vi "Dashboard Main.vi.BASE.11652.vi"() -> ()   [LabVIEW 2014]
uses:
  AutonModes.ctl
  <vilib>/event_ctls.llb/eventvkey.ctl
  <vilib>/Rock Robotics/WPI/Dashboard/WPI_DashboardLogging Global.vi
  <vilib>/Rock Robotics/Network Tables/SD Write String.vi
  <vilib>/Rock Robotics/Network Tables/SD Read String.vi
  <vilib>/Utility/config.llb/Write Key (String).vi
  <vilib>/Utility/config.llb/Write Key (I32).vi
  <vilib>/Utility/config.llb/NI_LVConfig.lvlib
panel:
  in  "TCP":refnum<k5>
  in  "Rec Mode":enum32{"Stop", "Record", "Playback"}(radio)
  in  "Vision":u16(ring) items=["Camera Off", "USB Camera SW", "USB Camera HW", "IP Camera"]
  out "Camera IP":string
  out "Image Message":string="Timeout in Camera Communications"
  in  "Dashboard Tab":T1(tab)
  in  "Camera Settings":T2={"Frame Rate"=30, "Compression"=30, "Size"=1} {"Frame Rate" scale=1.0..30.0; "Size" items=["640x480", "320x240", "160x120"]}
  out "MotorChart R":cluster{"Numeric":dbl, "Numeric":dbl}(graph)
  out "MotorChart L":T3(graph)
  out "MotorSliders R":cluster{"MotorSlide1":dbl, "MotorSlide2":dbl} {"MotorSlide2" scale=-1.0..1.0 scale format="%#_2e"; "MotorSlide1" scale=-1.0..1.0 scale format="%#_2e"}
  out "MotorSliders L":T4 {"MotorSlide4 2" scale=0.0..14.0 scale format="%#_2e"; "MotorSlide2" scale=-1.0..1.0 scale format="%#_2e"; "MotorSlide1" scale=-1.0..1.0 scale format="%#_2e"}
  out "Gyro":dbl(knob) scale=0.0..360.0
  out "JS1 Z":dbl(slide) scale=-1.0..1.0 scale format="%#_2e"
  out "JS1 Graph":cluster{"X":dbl, "Y":dbl}[](graph)
  out "JS1 Buttons":T5
  out "JS2 Z":dbl(slide) scale=-1.0..1.0 scale format="%#_2e"
  out "JS2 Graph":cluster{"X":dbl, "Y":dbl}[](graph)
  out "JS2 Buttons":T5
  out "Mode":T6(ring)=enum."Auto Disabled"
  in  "DB Camera Config":bool
  out "fps":dbl format="%#.1g"
  out "Mbps":dbl format="%#.1g"
  out "Mbps 2":bool
  in  "Open Config File":bool
  in  "Auton Mode":T7
  in  "Path to Auton Configs":path=path "C:/AutoConfig"
  out "Current Overdraw":bool
  out "Current":T8(graph)
  in  "DB/String 9":string
  in  "DB/String 8":string
  in  "DB/String 7":string
  in  "DB/String 6":string
  in  "DB/String 5":string
  in  "DB/String 4":string
  in  "DB/String 3":string
  in  "DB/String 2":string
  in  "DB/String 1":string
  in  "DB/String 0":string
  in  "DB/Slider 0":dbl(slide) scale=0.0..5.0
  in  "DB/Slider 1":dbl(slide) scale=0.0..5.0
  in  "DB/Slider 2":dbl(slide) scale=0.0..5.0
  in  "DB/Slider 3":dbl(slide) scale=0.0..5.0
  out "DB/LED 3":bool
  out "DB/LED 2":bool
  out "DB/LED 1":bool
  out "DB/LED 0":bool
  in  "DB/Button 3":bool
  in  "DB/Button 2":bool
  in  "DB/Button 1":bool
  in  "DB/Button 0":bool caption="New Name"
  in  "Test Slider":dbl(slide) scale=0.0..100.0 scale format="%#_3g"
  in  "On/Off":bool caption="Solenoid"
  in  "Test Name":u16(ring) items=["Select the test to run...", "Example Test", "-------------------------------", "List of tests is built in robot code.", "Replace with your own automated tests."]
  in  "Test Tree":string(tree)
  in  "Motor":cluster{"Value":dbl, "Enable":bool} {"Value" scale=-1.0..1.0 scale format="%#_3g"}
  out "Progress":T9 {"Test Progress" scale=0.0..100.0}
  in  "Rev/Fwd":cluster{"Forward":bool, "Reverse":bool}
  in  "Test Ring":u16(ring) items=["Monochrome", "Color"]
  in  "Listbox":i32(listbox)
  out "Tree":string(tree)
  out "Camera Image":T10(plugin-control)
  out "Boolean":bool
  # "Left"
  # "Front"
  # "Right"
  # "Battery"
  # "This tab is a great place for autonomous settings and robot-specific values.\nPlace controls and indicators inside this tab and match name to\nDashboard Variables on robot. You can also delete this comment."
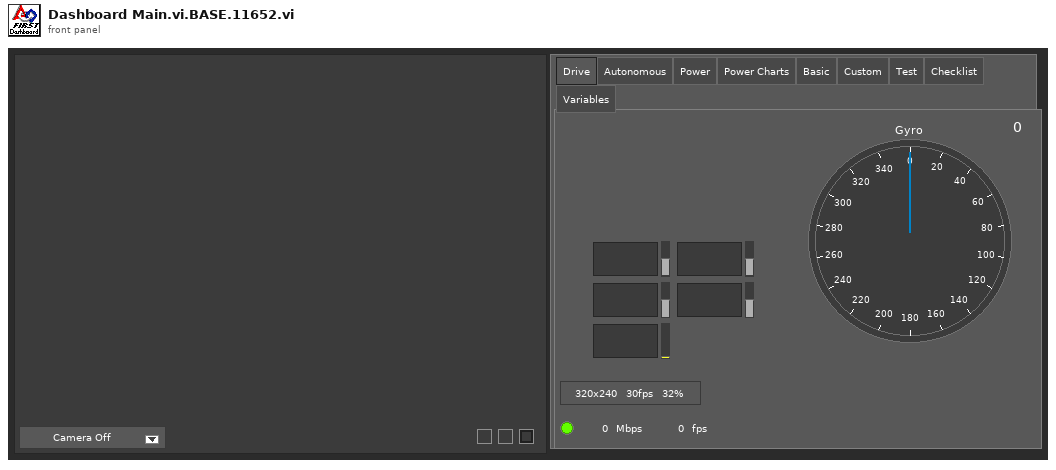
[diagram p1: front panel]
types:
  T1 = enum32{"Drive", "Autonomous", "Power", "Power Charts", "Basic", "Custom", "Test", "Checklist", "Variables"}
  T2 = cluster{"Frame Rate":i32, "Compression":i32, "Size":u16}
  T3 = cluster{"Numeric":dbl, "Numeric":dbl, "Battery V":dbl}
  T4 = cluster{"MotorSlide1":dbl, "MotorSlide2":dbl, "MotorSlide4 2":dbl}
  T5 = cluster{bool, bool, bool, bool, bool, bool, bool, bool, bool, bool, bool, bool}
  T6 = enum8{"Tele-Op Disabled", "Tele-Op Enabled", "Auto Disabled", "Auto Enabled", "Test Disabled", "Test Enabled", "Disconnected", "No Code", "E-Stop"}
  T7 = typedef "AutonModes.ctl" = enum32{"Sit Still", "Go Get That Tote!", "Custom 1", "Custom 2", "FromLandfill", "CanGrab"}
  T8 = cluster{"Numeric":dbl, "Numeric":dbl, "Numeric":dbl, "Numeric":dbl, "Numeric":dbl}
  T9 = cluster{"Test Progress":u8, "Test Progress Text":string}
  T10 = typedef "IMAQ Image.ctl" = refnum<image>
  T11 = enum32{"Drive", "Basic", "Custom", "Test", "Checklist", "Variables"}
  T12 = typedef "Image Type" = u32
  T13 = cluster{"Camera Image":refnum<vi>, "Dashboard Tab":refnum<vi>, "Boolean":refnum<vi>, "Vision":refnum<vi>, "Rec Mode":refnum<vi>, "Test Slider":refnum<vi>, "On/Off ":refnum<vi>, "Test Ring":refnum<vi>, "Rev/Fwd":refnum<vi>, "Test Name":refnum<vi>, "Motor":refnum<vi>, "Progress":refnum<vi>, "CheckList":refnum<vi>, "Tree":refnum<vi>, "Test Tree":refnum<vi>}
  T14 = enum16{"open", "replace", "create", "open or create", "replace or create", "replace or create with confirmation"}
  T15 = cluster{"Error Strings":string, "Disable Counts":cluster{u16, u16}, "Rail Faults":cluster{u16, u16, u16}, "Robot IP":string, "DB Mode":u8, "Event Info":cluster{"Name":string, "Type":u8, "Number":u16, "Replay":u8}, "Camera Addr":string}
  T16 = cluster{"Storage":cluster{"Disk Free":u64, "RAM Block":u32, "RAM free":u32}, "CPU Utilization":cluster{"CPU % ISR":sgl, "CPU % Time Crit":sgl, "CPU % Timed Str":sgl, "CPU % High":sgl, "CPU % Above":sgl, "CPU % Normal":sgl, "CPU % Low":sgl}, "CAN":cluster{"% Bus Utilization":sgl, "Bus Off Cnt":u32, "TX_FIFO Full Cnt":u32, "Receive Error Cnt":u8, "Transmit Error Cnt":u8}, "HID":cluster{"HID Outputs":u32, "Rumble Low":u16, "Rumble High":u16}[]}
  T17 = cluster{"Status bits":cluster{"Test Mode":bool, "Autonomous":bool, "Enabled":bool, "Code Start":bool, "Brownout":bool, "Reserved 2":bool, "Reserved 3":bool, "E-Stop":bool}, "Code Trace":cluster{"Disabled":bool, "TeleOp":bool, "Auto":bool, "Test":bool}, "Controller Type":enum16{"unknown", "cRIO", "roboRio"}, "Code?":enum16{"unknown", "noCode", "code"}, "Battery V":dbl}
  T18 = cluster{"Control Bits":cluster{"TestMode":bool, "Autonomous":bool, "Enabled":bool, "FMS Present":bool, bool, bool, bool, "E-Stop":bool}, "Team Station ":u8, "Countdown":sgl, "Joystick Values":cluster{"Axes":dbl[], "Buttons":bool[], "POVs":i16[]}[]}
  T19 = cluster{"Axes":dbl[], "Buttons":bool[], "POVs":i16[]}[]
  T20 = cluster{"Axes":dbl[], "Buttons":bool[], "POVs":i16[]}
  T21 = cluster{"Buttons[0]":bool, "Buttons[1]":bool, "Buttons[2]":bool, "Buttons[3]":bool, "Buttons[4]":bool, "Buttons[5]":bool, "Buttons[6]":bool, "Buttons[7]":bool, "Buttons[8]":bool, "Buttons[9]":bool, "Buttons[10]":bool, "Buttons[11]":bool}
  T22 = typedef "NI_LVConfig.lvlib/Config Data RefNum.ctl" = refnum<k1>
  T23 = cluster{"Operation":enum16{"Update", "Clear"}, "Color Box":u32}[]
  T24 = typedef "eventvkey.ctl" = enum16{"ASCII", "Enter", "Return", "Shift", "Ctrl", "Alt", "Cmd", "Opt", "Caps", "NumLock", "Clear", "Break", "Up", "Down", "Left", "Right", "Insert", "Delete", "Home", "End", "PageUp", "PageDown", "Escape", "Help", "Pause", "ScrollLock", "F1", "F2", "F3", "F4", "F5", "F6", "F7", "F8", "F9", "F10", "F11", "F12", "F13", "F14", "F15", "F16", "F17", "F18", "F19", "F20", "F21", "F22", "F23", "F24", "Play", "VolumeUp", "VolumeDown", "Mute", "Two Byte Char"}
  T25 = cluster{"Image Size":bool, "Image Type":bool, "Pixel Value":bool, "ROI Information":bool, "Zoom Factor":bool}
  T26 = enum8{"Enabled", "Disabled", "Disabled and Grayed Out"}
  T27 = cluster{"Operation":enum16{"Update", "Clear"}, "Color Box":u32}
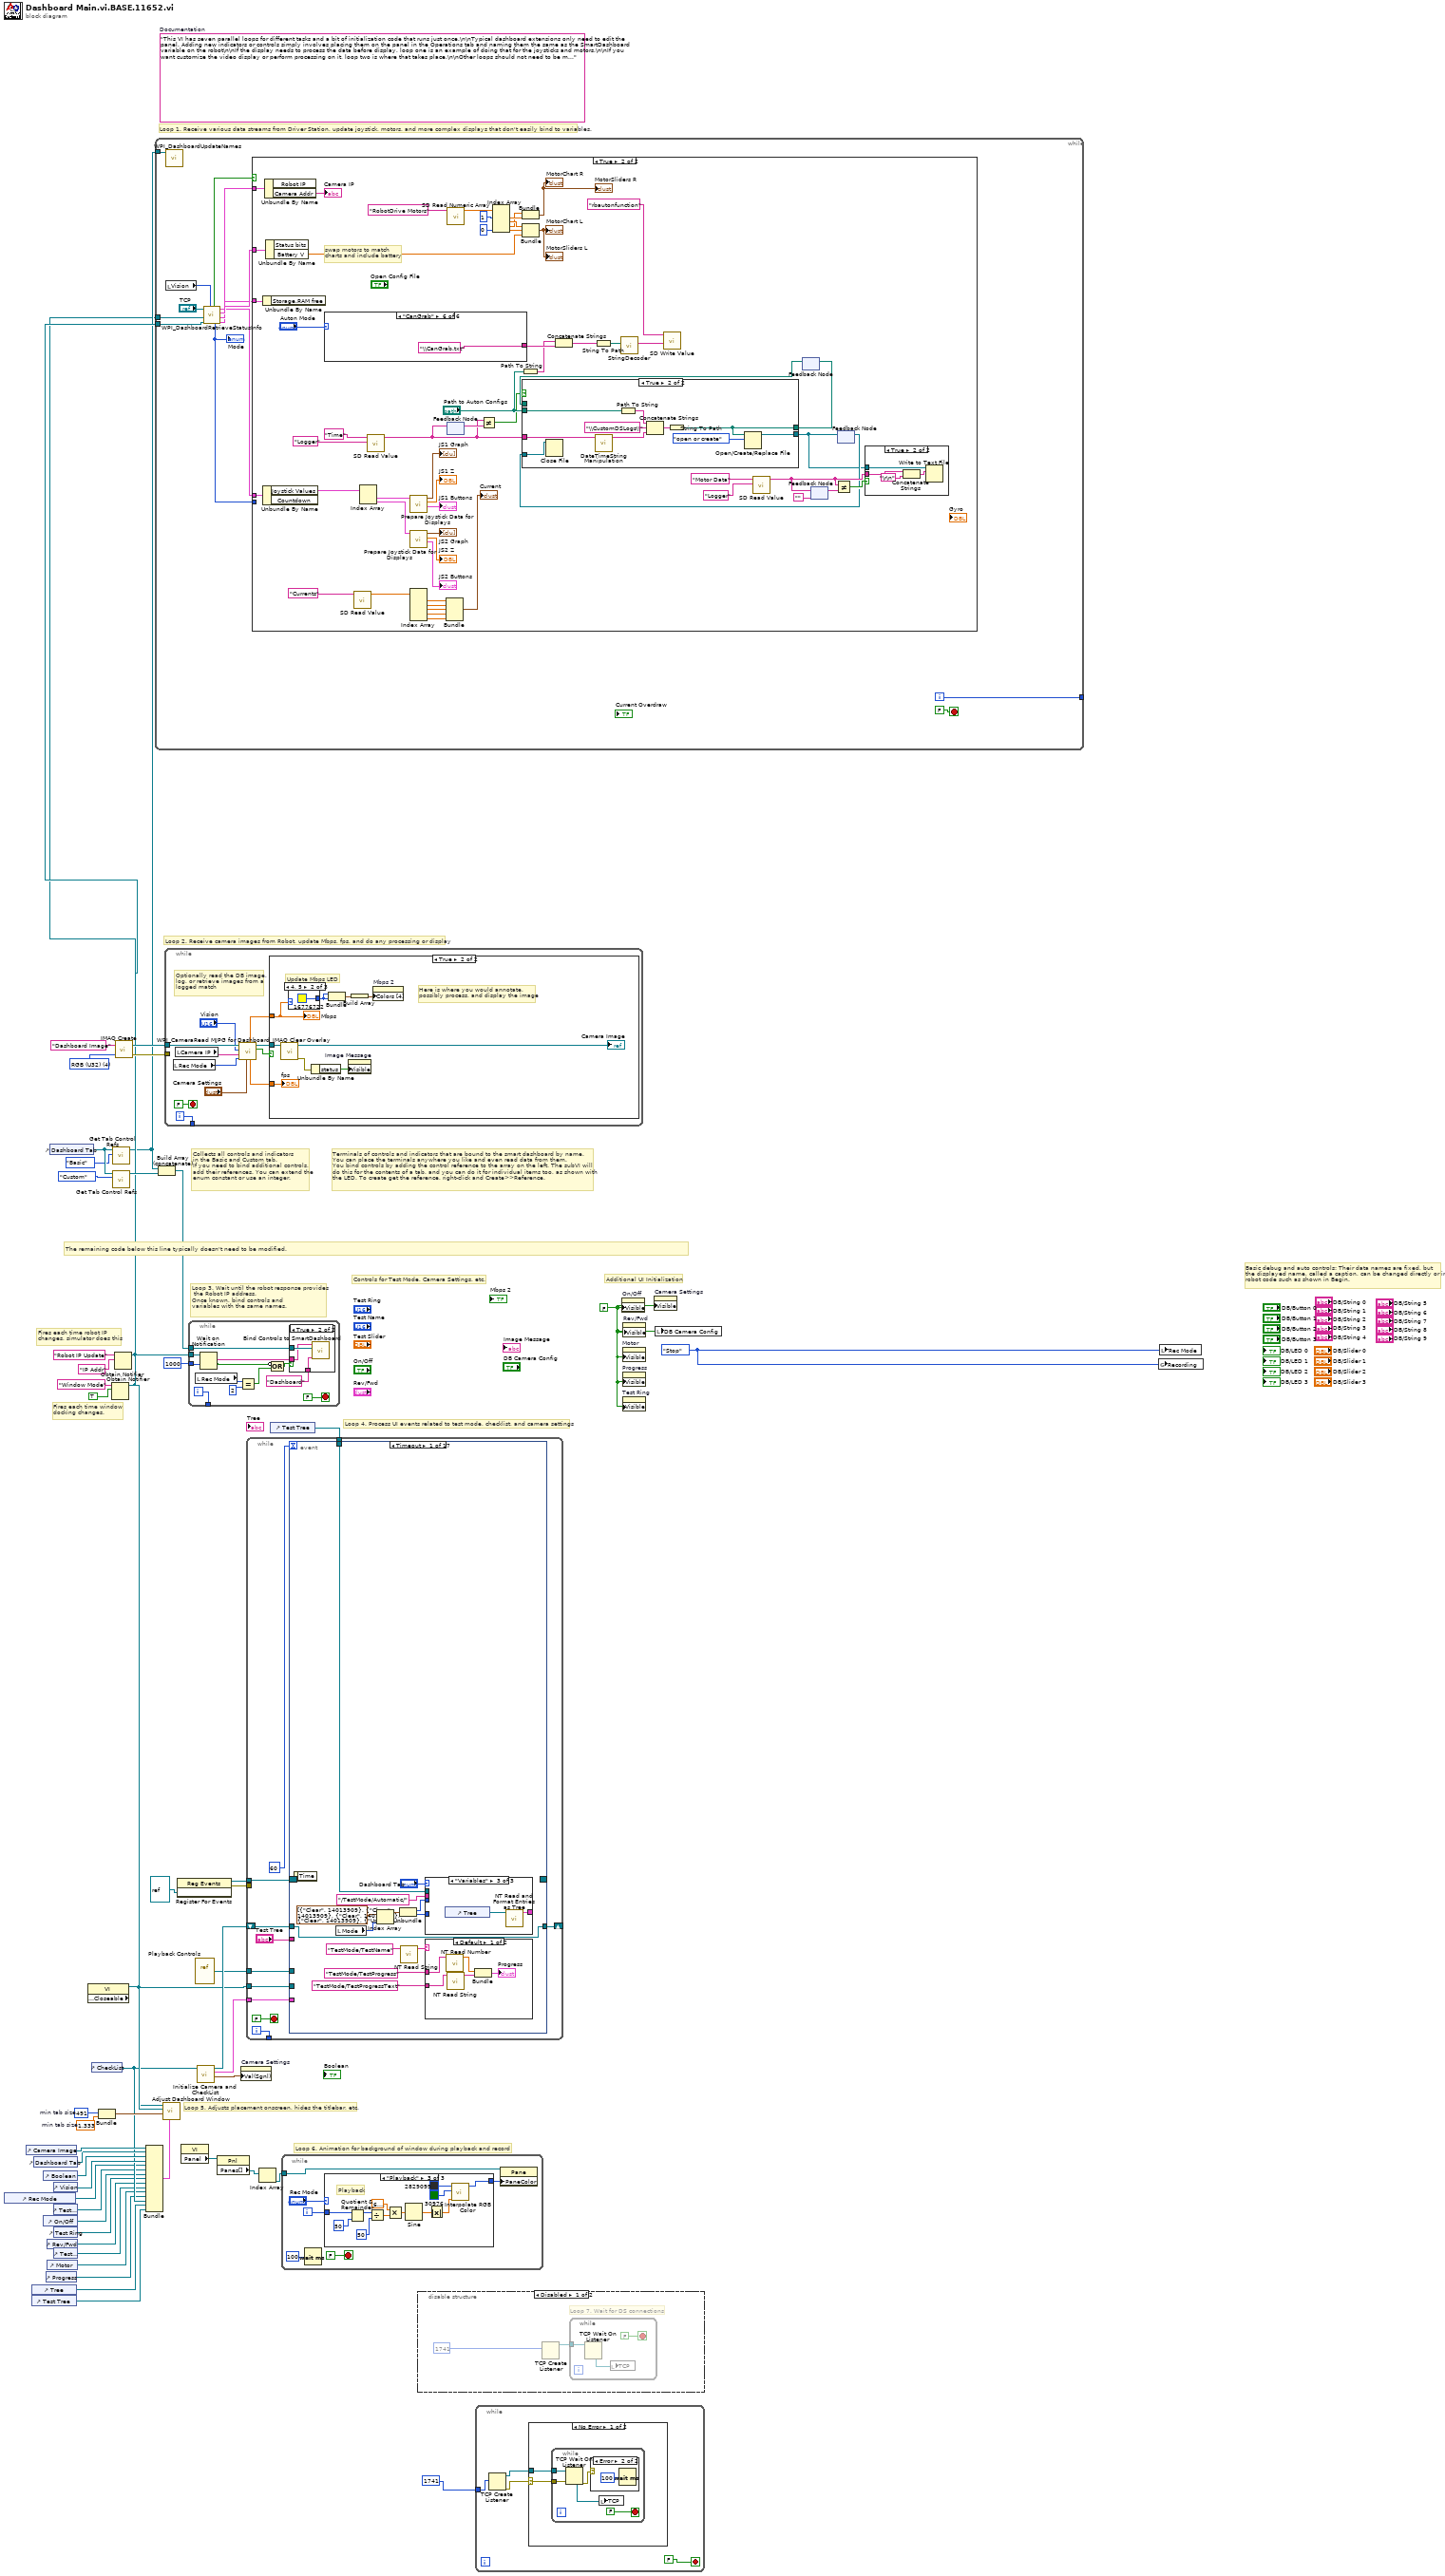
[diagram p0: block diagram]
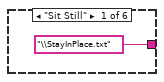
[diagram p8: hidden frame]
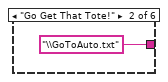
[diagram p9: hidden frame]
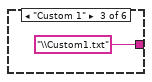
[diagram p10: hidden frame]
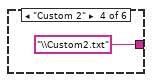
[diagram p11: hidden frame]
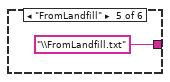
[diagram p12: hidden frame]
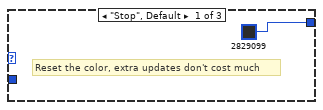
[diagram p13: hidden frame]
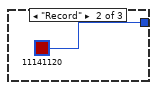
[diagram p14: hidden frame]
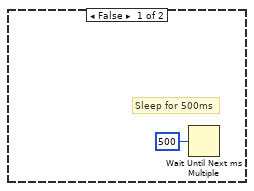
[diagram p16: hidden frame]
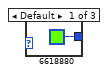
[diagram p17: hidden frame]
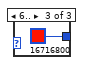
[diagram p18: hidden frame]
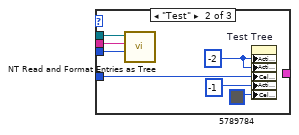
[diagram p20: hidden frame]
diagram:
  w23 = 491  # min tab size
  w22 = 1.333  # min tab size
  w31 = enum32{"Stop", "Record", "Playback"}."Stop" ("Rec Mode")
  w5 = FALSE ("Visible")
  (unwired) "This VI has seven parallel loops for different tasks and a bit of initialization code that runs just once.\n\nTypical dashboard extensions only need to edit the panel. Adding new indicators or controls simply involves placing them on the panel in the Operations tab and naming them the same as the SmartDashboard variable on the robot\n\nIf the display needs to process the data before display, loop one is an example of doing that for the joysticks and motors.\n\nIf you want customize the video display or perform processing on it, loop two is where that takes place.\n\nOther loops should not need to be modified. They are pretty standard, and document the task they perform."  # Documentation
  w51 = T12 4 items=["Grayscale (U8)", "Grayscale (I16)", "Grayscale (SGL)", "Complex (CSG)", "RGB (U32)", "HSL (U32)", "RGB (U64)"] ("Image Type")
  # "Basic debug and auto controls: Their data names are fixed, but\nthe displayed name, called a caption, can be changed directly or in\nrobot code such as shown in Begin."
  # "Controls for Test Mode, Camera Settings, etc."
  # "Additional UI Initialization"
  # "Loop 6. Animation for background of window during playback and record"
  # "Fires each time robot IP\nchanges, simulator does this"
  # "Fires each time window\ndocking changes."
  # "Collects all controls and indicators\nin the Basic and Custom tab.\nIf you need to bind additional controls,\nadd their references. You can extend the\nenum constant or use an integer."
  # "The remaining code below this line typically doesn't need to be modified."
  # "Loop 4. Process UI events related to test mode, checklist, and camera settings"
  # "Terminals of controls and indicators that are bound to the smart dashboard by name.\nYou can place the terminals anywhere you like and even read data from them.\nYou bind controls by adding the control reference to the array on the left. The subVI will\ndo this for the contents of a tab, and you can do it for individual items too, as shown with\nthe LED. To create get the reference, right-click and Create>>Reference."
  # "Loop 3. Wait until the robot response provides\n the Robot IP address.\nOnce known, bind controls and\nvariables with the same names."
  # "Loop 5. Adjusts placement onscreen, hides the titlebar, etc."
  # "Loop 1. Receive various data streams from Driver Station, update joystick, motors, and more complex displays that don't easily bind to variables."
  # "Loop 2. Receive camera images from Robot, update Mbps, fps, and do any processing or display"
  n1 = control-ref of="Rec Mode"() -> (w11:refnum<vi>)
  n2 = control-ref of="Camera Image"() -> (w26:refnum<vi>)
  n3 = control-ref of="Tree"() -> (w15:refnum<vi>)
  n4 = control-ref of="Test Tree"() -> (w14:refnum<vi>)
  n5 = control-ref of="Dashboard Tab"() -> (w25:refnum<vi>)
  n6 = control-ref of="Boolean"() -> (w20:refnum<vi>)
  n7 = control-ref of="On/Off"() -> (w9:refnum<vi>)
  n8 = control-ref of="Progress"() -> (w6:refnum<vi>)
  n9 = control-ref of="Rev/Fwd"() -> (w7:refnum<vi>)
  n10 = control-ref of="Motor"() -> (w12:refnum<vi>)
  n11 = control-ref of="Dashboard Tab"() -> (w29:refnum<vi>)
  n12 = control-ref of="Test Slider"() -> (w10:refnum<vi>)
  n13 = control-ref of="Vision"() -> (w24:refnum<vi>)
  n14 = control-ref of="Test Ring"() -> (w8:refnum<vi>)
  n15 = control-ref of="Test Name"() -> (w13:refnum<vi>)
  n16 = property class="VI" props=["Front Panel.Closeable"]() -> (reference out=w30:refnum<vi>)  [unwired: 2 in, 2 out]
  n17 = control-ref of="CheckList"() -> (w16:refnum<vi>)
  n18 = Bundle("min tab size"=w23, "min tab size"=w22) -> (w21:cluster{"min tab size":i32, "min tab size":dbl})  [unwired: 1 in]
  n19 = Obtain Notifier(name (unnamed)="Window Mode", notification data type=TRUE) -> (notifier out=w2:refnum<notifier>)  [unwired: 2 in, 2 out]
  n20 = call <vilib>:"Get Tab Control Refs.vi"("Page Index"=T11."Basic" ("Dashboard Tab"), "TabControl in"=w29) -> ("ControlsOnPage"=w3:refnum<vi>[])  [unwired: 9 in]
  n21 = call <vilib>:"Get Tab Control Refs.vi"("Page Index"=T11."Custom" ("Dashboard Tab"), "TabControl in"=w29) -> ("ControlsOnPage"=w28:refnum<vi>[])  [unwired: 9 in]
  n22 = Obtain Notifier(name (unnamed)="Robot IP Update", notification data type="IP Addr" ("name (unnamed)")) -> (notifier out=w4:refnum<notifier>)  [unwired: 2 in, 2 out]
  n23 = call "IMAQ Create"("Image Name"="Dashboard Image", "Image Type"=w51) -> ("New Image"=w49:T10, "error out"=w48:errorcluster)  [unwired: 2 in, 1 out]
  n24 = Bundle("Camera Image"=w26, "Dashboard Tab"=w25, "Boolean"=w20, "Vision"=w24, "Rec Mode"=w11, "Test Slider"=w10, "On/Off"=w9, "Test Ring"=w8, "Rev/Fwd"=w7, "Test Name"=w13, "Motor"=w12, "Progress"=w6, "CheckList"=w16, "Tree"=w15, "Test Tree"=w14) -> (w17:T13)  [unwired: 1 in]
  n25 = while {
    tunnel: [w63] -> _
    tunnel: w4 -> [w57]
    tunnel: w3 -> [w56]
    tunnel: w2 -> [w52]
    i -> [w63]
    stop <- FALSE stop-if-true
    n26 = call <vilib>:"WPI_DashboardUpdateNames.vi"("Controls on Tab"=w56) -> ()  [unwired: 11 in]
    n27 = local read "Vision"() -> (w54:u16)
    n28 = call <vilib>:"WPI_DashboardRetrieveStatusInfo.vi"("Vision"=w54, "Binding Refnum"=w57, "Window Mode Notifier"=w52, "TCP Cnx"="TCP") -> ("Power and Errors"=w58:T15, "Robot Metrics"=w61:T16, "Status Info"=w62:T17, "Control Info"=w59:T18, "Robot Mode"=w55:T6, "Process?"=w60:bool)  [unwired: 2 in]
    "Mode" <- w55
    n29 = case shown="True" w60 {
      tunnel: w62 -> [_ w120]
      tunnel: w61 -> [_ w119]
      tunnel: w59 -> [_ w118]
      tunnel: w58 -> [_ w117]
      tunnel: w55 -> [_ _]
      frame False {
      }
      frame True {
        # "swap motors to match\ncharts and include battery"
        n30 = Unbundle By Name(w119) -> ()  [unwired: 1 out]
        n31 = Unbundle By Name(w118) -> ("Joystick Values"=w105:T19)  [unwired: 1 out]
        n32 = Unbundle By Name(w117) -> ("Camera Addr"=→"Camera IP":string)  [unwired: 1 out]
        n33 = Unbundle By Name(w120) -> ("Battery V"=w106:dbl)  [unwired: 1 out]
        n34 = case shown="\"CanGrab\"" "Auton Mode" {
          tunnel: ["\\StayInPlace.txt" "\\GoToAuto.txt" "\\Custom1.txt" "\\Custom2.txt" "\\FromLandfill.txt" "\\CanGrab.txt"] -> w84
          frame "Sit Still" {
          }
          frame "Go Get That Tote!" {
          }
          frame "Custom 1" {
          }
          frame "Custom 2" {
          }
          frame "FromLandfill" {
          }
          frame "CanGrab" {
          }
        }
        n35 = call-poly <vilib>:"SD Read Value.vi"("Name"="Currents") -> ("Numeric Array"=w91:dbl[])  [unwired: 8 in, 2 out]
        n36 = Index Array(array=w105) -> (element #1=w104:T20, element #2=w99:T20)  [unwired: 2 in]
        n37 = call-poly <vilib>:"SD Read Value.vi"("Table Prefix"="Logger", "Name"="Time") -> ("String"=w67:string)  [unwired: 7 in, 2 out]
        n38 = call "Prepare Joystick Data for Displays.vi"("Joystick Values"=w104) -> ("Buttons"=→"JS1 Buttons":T21, "Z Axis"=→"JS1 Z":dbl, "Cartesian Data"=→"JS1 Graph":cluster{"X axis":dbl, "X axis":dbl}[])  [unwired: 8 in]
        n39 = call "Prepare Joystick Data for Displays.vi"("Joystick Values"=w99) -> ("Buttons"=→"JS2 Buttons":T21, "Z Axis"=→"JS2 Z":dbl, "Cartesian Data"=→"JS2 Graph":cluster{"X axis":dbl, "X axis":dbl}[])  [unwired: 8 in]
        n40 = Index Array(array=w91) -> (element #1=w90:dbl, element #2=w89:dbl, element #3=w88:dbl, element #4=w87:dbl, element #5=w86:dbl)  [unwired: 5 in]
        n41 = Bundle("Numeric"=w90, "Numeric"=w89, "Numeric"=w88, "Numeric"=w87, "Numeric"=w86) -> (→"Current":T8)  [unwired: 1 in]
        n42 = call <vilib>:"SD Read Numeric Array.vi"("Name"="RobotDrive Motors") -> ("Numeric Array"=w108:dbl[])  [unwired: 8 in, 2 out]
        n43 = feedback #1() -> (w69:string)  [unwired: 1 in]
        n44 = feedback-in #1(w67) -> ()
        n45 = Not Equal?(x=w67, y=w69) -> (x != y?=w68:bool)
        n46 = Index Array(array=w108, index #1=1, index #4=0) -> (element #1=w112:dbl, element #2=w113:dbl, element #3=w111:dbl, element #4=w116:dbl)  [unwired: 2 in]
        n47 = Path To String(path="Path to Auton Configs") -> (string=w83:string)
        n48 = Bundle("Numeric"=w111, "Numeric"=w112) -> (→"MotorChart R" →"MotorSliders R":cluster{"Numeric":dbl, "Numeric":dbl})  [unwired: 1 in]
        n49 = Bundle("Numeric"=w113, "Numeric"=w116, "Battery V"=w106) -> (→"MotorChart L" →"MotorSliders L":T3)  [unwired: 1 in]
        n50 = Concatenate Strings(w83, w84) -> (w82:string)
        n51 = String To Path(string=w82) -> (path=w81:path)
        n52 = call "StringDecoder.vi"("Auto Config File"=w81) -> ("RobotDataString"=w94:string)  [unwired: 10 in]
        n53 = call-poly <vilib>:"SD Write Value.vi"("String"=w94, "Name"="rbautonfunction") -> ()  [unwired: 8 in, 2 out]
        n54 = call-poly <vilib>:"SD Read Value.vi"("Table Prefix"="Logger", "Name"="Motor Data") -> ("String"=w75:string)  [unwired: 7 in, 2 out]
        n55 = feedback #2() -> (w72:path)  [unwired: 1 in]
        n56 = feedback-in #3(w75) -> ()
        n57 = feedback #3("") -> (w77:string)
        n58 = Not Equal?(x=w75, y=w77) -> (x != y?=w76:bool)
        n59 = feedback #4() -> (w66:refnum<file>)  [unwired: 1 in]
        n60 = case shown="True" w68 {
          tunnel: [w122 w124] -> w73
          tunnel: "Path to Auton Configs" -> [_ w128]
          tunnel: w72 -> [w122 _]
          tunnel: w67 -> [_ w127]
          tunnel: [w121 w125] -> w65
          tunnel: w66 -> [w121 w123]
          frame False {
          }
          frame True {
            n61 = Close File(refnum=w123) -> ()  [unwired: 1 in, 2 out]
            n62 = call "DateTimeString Manipulation.vi"("FPU DT String"=w127) -> ("FPF DT String"=w132:string)  [unwired: 4 in]
            n63 = Path To String(path=w128) -> (string=w130:string)
            n64 = Concatenate Strings(w130, "\\CustomDSLogs\\", w132) -> (w129:string)
            n65 = String To Path(string=w129) -> (path=w124:path)
            n66 = Open/Create/Replace File(file path (use dialog)=w124, operation (0:open)=T14."open or create") -> (refnum out=w125:refnum<file>)  [unwired: 4 in, 2 out]
          }
        }
        n67 = feedback-in #2(w73) -> ()
        n68 = feedback-in #4(w65) -> ()
        n69 = case shown="True" w76 {
          tunnel: w75 -> [_ w135]
          tunnel: w65 -> [_ w133]
          frame False {
          }
          frame True {
            n70 = Concatenate Strings(w135, "\r\n") -> (w134:string)
            n71 = Write to Text File(file (use dialog)=w133, text=w134) -> ()  [unwired: 2 in, 3 out]
          }
        }
      }
    }
  }
  n72 = Build Array (concatenate)(w3, w28) -> (w27:refnum<vi>[])
  n73 = call "Adjust Dashboard Window.vi"("Sizing Refnums"=w17, "Size Constraints"=w21, "VI"=w30, "Notifier in"=w2) -> ()  [unwired: 8 in]
  n74 = while {
    tunnel: w49 -> [w151]
    tunnel: w48 -> [_]
    tunnel: [w152] -> _
    i -> [w152]
    stop <- FALSE stop-if-true
    # "Optionally read the DB image,\nlog, or retrieve images from a\nlogged match"
    n75 = local read "Rec Mode"() -> (w145:enum32{"Stop", "Record", "Playback"})
    n76 = local read "Camera IP"() -> (w143:string)
    n77 = call <vilib>:"WPI_CameraRead MJPG for Dashboard.vi"("Camera Settings"="Camera Settings", "Rec Mode"=w145, "Camera IP"=w143, "Camera Mode"="Vision", "Refnum in"=w151) -> ("Active"=w149:bool, "Refnum out"=w150:T10, "FPS"=w148:dbl, "Bandwidth (Mbps)"=w147:dbl)  [unwired: 3 in]
    n78 = case shown="True" w149 {
      tunnel: w150 -> [_ w158]
      tunnel: w147 -> [_ w157]
      tunnel: w148 -> [_ w155]
      frame False {
        # "Sleep for 500ms"
        n79 = Wait Until Next ms Multiple(millisecond multiple=u32 500) -> ()  [unwired: 1 out]
      }
      frame True {
        # "Here is where you would annotate,\npossibly process, and display the image"
        # "Update Mbps LED"
        n80 = call "IMAQ Clear Overlay"("Image"=w158) -> ("error out"=w162:errorcluster, "Image Out"=→"Camera Image":T10)  [unwired: 2 in, 7 out]
        n81 = case shown="4, 5" w157 {
          tunnel: [u32 6618880 ("Color Box") u32 16776722 ("Color Box") u32 16716800 ("Color Box")] -> w159
          frame Default {
          }
          frame 4, 5 {
          }
          frame 6.. {
          }
        }
        n82 = Unbundle By Name(w162) -> ("status"=w163:bool)
        n83 = Bundle("Color Box"=w159, "Color Box"=w159) -> (w161:cluster{"Color Box":u32, "Color Box":u32})  [unwired: 1 out]
        n84 = property on="Image Message" class="Str"("Visible"=w163) -> ()  [unwired: 2 in, 2 out]
        n85 = Build Array(w161) -> (w160:cluster{"Color Box":u32, "Color Box":u32}[])
        n86 = property on="Mbps 2" class="Bool (strict)"("Colors [4]"=w160) -> ()  [unwired: 2 in, 2 out]
        "Mbps" <- w157
        "fps" <- w155
      }
    }
  }
  n87 = register-events(refnum<vi> refnum) -> (reference out=w35:refnum<event-registration>, error out=w34:errorcluster)  [unwired: 2 in]
  n88 = property class="VI"() -> ("Panel"=w38:refnum<vi>)  [unwired: 2 in, 2 out]
  n89 = while {
    tunnel: w27 -> [w178]
    tunnel: w4 -> [w176]
    tunnel: [w174] -> _
    tunnel: u32 1000 ("milliseconds to wait") -> [w173]
    i -> [w174]
    stop <- FALSE stop-if-true
    n90 = local read "Rec Mode"() -> (w169:enum32{"Stop", "Record", "Playback"})
    n91 = Wait on Notification(notifier=w176, timeout in ms (-1)=w173) -> (notification=w175:string, timed out?=w171:bool)  [unwired: 2 in, 2 out]
    n92 = Equal?(x=w169, y=u16 2 ("Rec Mode")) -> (x = y?=w170:bool)
    n93 = Compound Arithmetic op=OR(invert w171, w170) -> (w172:bool)
    n94 = case shown="True" w172 {
      tunnel: w178 -> [_ w181]
      tunnel: w175 -> [_ w180]
      tunnel: "Dashboard" -> [_ w179]
      frame False {
      }
      frame True {
        n95 = call <vilib>:"Bind Controls to SmartDashboard.vi"("Client Name"=w179, "Bound Control Refs"=w181, "Server IP Address"=w180) -> ()  [unwired: 9 in]
      }
    }
  }
  n96 = vi-ref "Playback Controls.vi"() -> (w36:refnum<vi>)
  n97 = call "Initialize Camera and CheckList.vi"("ListBox in"=w16) -> ("Cluster"=w42:cluster{"value":i32, "value":i32, "index":i32}, "Array"=w43:cluster{string[]}[], "File Refnum"=w41:T22)  [unwired: 8 in]
  n98 = property class="Pnl"(reference=w38) -> ("Panes[]"=w39:refnum<vi>[])  [unwired: 1 in, 2 out]
  n99 = property on="Camera Settings" class="Clust (strict)"("Val(Sgnl)"=w42) -> ()  [unwired: 2 in, 2 out]
  n100 = Index Array(array=w39) -> (element=w37:refnum<vi>)  [unwired: 1 in]
  n101 = control-ref of="Test Tree"() -> (w40:refnum<vi>)
  n102 = while {
    tunnel: w43 -> [w189]
    shift-right: [w188] -> _
    shift-left: w41 -> [w187]
    tunnel: [w186] -> _
    tunnel: w40 -> [w185]
    tunnel: w36 -> [w184]
    tunnel: w35 -> [w183]
    tunnel: w34 -> [_]
    tunnel: w30 -> [w182]
    i -> [w186]
    stop <- FALSE stop-if-true
    n103 = event shown="[0] Timeout" {
      selector: w183 -> [_ _ _ _ _ _ _ _ _ _ _ _ _ _ _ _ _]
      dyn-events: [_ _ _ _ _ _ _ _ _ _ _ _ _ w427 _ _ _] -> _
      timeout: u32 60 ("milliseconds to wait") -> [_ _ _ _ _ _ _ _ _ _ _ _ _ _ _ _ _]
      tunnel: w185 -> [w201 _ _ _ _ _ _ _ _ _ _ _ _ _ _ _ _]
      tunnel: "Test Tree" -> [_ _ _ _ _ _ _ _ w396 w404 w406 w410 w418 _ _ _ _]
      tunnel: w189 -> [_ w223 _ _ _ _ w360 w390 _ _ _ _ _ _ _ _ _]
      tunnel: [w197 w222 w321 w326 w334 w346 w359 w383 w395 w402 w405 w409 w417 w429 w443 w444 w454] -> w188
      tunnel: w187 -> [w197 w222 w321 w326 w334 w346 w358 w383 w395 w402 w405 w409 w417 w429 w443 w444 w454]
      tunnel: w184 -> [_ _ _ _ _ _ _ _ _ _ _ _ _ w430 _ w447 _]
      tunnel: w182 -> [_ _ _ _ _ _ _ _ _ _ _ _ _ w425 _ _ _]
      event Timeout {
        n104 = event-data() -> ()  [unwired: 1 in, 1 out]
        n105 = local read "Mode"() -> (w200:T6)
        n106 = Index Array(array=T23 [{"Operation"=enum."Clear", "Color Box"=14013909}, {"Operation"=enum."Clear", "Color Box"=14013909}, {"Operation"=enum."Clear", "Color Box"=14013909}, {"Operation"=enum."Clear", "Color Box"=14013909}, {"Operation"=enum."Update", "Color Box"=14013909}, {"Operation"=enum."Update", "Color Box"=16777215}, {"Operation"=enum."Clear", "Color Box"=14013909}, {"Operation"=enum."Clear", "Color Box"=14013909}, {"Operation"=enum."Clear", "Color Box"=14013909}], index=w200) -> (element=w195:T27)
        n107 = Unbundle(w195) -> ("Operation"=w194:enum16{"Update", "Clear"}, "Color Box"=w193:u32)
        n108 = call <vilib>:"NT Read String.vi"("Name"="TestMode/TestName") -> ("String"=w204:string)  [unwired: 9 in, 1 out]
        n109 = case shown="\"Variables\"" "Dashboard Tab" {
          tunnel: w201 -> [_ w212 _]
          tunnel: "/TestMode/Automatic/" ("Name Pattern") -> [_ w211 _]
          tunnel: w194 -> [_ w210 _]
          tunnel: [_ _ w214] -> _
          tunnel: w193 -> [_ w206 _]
          frame "Custom", Default {
          }
          frame "Test" {
            w209 = -2 ("Active Item:Row Number")
            n110 = call <vilib>:"NT Read and Format Entries as Tree.vi"("Operation"=w210, "Name Pattern"=w211, "Tree Refnum"=w212) -> ()  [unwired: 7 in, 2 out]
            n111 = property on="Test Tree" class="Tree (strict)"("Active Item Row Number"=w209, "ActiveColNum"=w209, "CellBG"=w206, "Active Item Row Number"=-1 ("Active Item:Row Number"), "CellBG"=u32 5789784 ("Color Box")) -> ()  [unwired: 2 in, 2 out]
          }
          frame "Variables" {
            n112 = control-ref of="Tree"() -> (w213:refnum<vi>)
            n113 = call <vilib>:"NT Read and Format Entries as Tree.vi"("Tree Refnum"=w213) -> ("Formatted Strings"=w214:cluster{"Name":string, "Value":string}[])  [unwired: 9 in, 1 out]
          }
        }
        n114 = case shown="Default" w204 {
          tunnel: "TestMode/TestProgress" ("Name") -> [w216 _]
          tunnel: "TestMode/TestProgressText" ("Name") -> [w215 _]
          frame Default {
            n115 = call <vilib>:"NT Read Number.vi"("Name"=w216) -> ("Numeric"=w217:dbl)  [unwired: 9 in, 1 out]
            n116 = call <vilib>:"NT Read String.vi"("Name"=w215) -> ("String"=w218:string)  [unwired: 9 in, 1 out]
            n117 = Bundle("Numeric"=w217, "String"=w218) -> (→"Progress":cluster{"Numeric":dbl, "String":string})  [unwired: 1 in]
          }
          frame "" {
            n118 = property on="Progress" class="Clust (strict)"("Visible"=FALSE) -> ()  [unwired: 2 in, 2 out]
            n119 = local write "Test Name"(u16 0) -> ()
          }
        }
      }
      event "Test Tree": Value Change {
        # "Show appropriate\ncontrols"
        n120 = event-data() -> ("CtlRef"=w226:refnum<vi>, "NewVal"=w224:string)  [unwired: 1 in]
        n121 = call <vilib>:"WPI_UtilitiesGetTreeIOName.vi"("NewVal"=w224, "TreeControl in"=w226) -> ("I/O Name"=w227:string)  [unwired: 9 in]
        n122 = case shown="\"Camera\"" w227 {
          selector: w227 -> [_ w234 _ w252 w261 _]
          tunnel: w224 -> [_ _ w249 w251 _ w268]
          tunnel: w223 -> [_ _ _ _ _ w267]
          frame Default {
            w229 = FALSE ("Visible")
            w228 = FALSE ("Visible")
            n123 = property on="Motor" class="Clust (strict)"("Visible"=w228) -> ()  [unwired: 2 in, 2 out]
            n124 = property on="Test Ring" class="Ring (strict)"("Visible"=w228) -> ()  [unwired: 2 in, 2 out]
            n125 = property on="Rev/Fwd" class="Clust (strict)"("Visible"=w229) -> ()  [unwired: 2 in, 2 out]
            n126 = property on="On/Off" class="Bool (strict)"("Visible"=w229) -> ()  [unwired: 2 in, 2 out]
            n127 = property on="Test Slider" class="Slide (strict)"("Visible"=w229) -> ()  [unwired: 2 in, 2 out]
          }
          frame "Motor", "PWM" {
            w235 = FALSE ("Visible")
            n128 = case shown="\"Motor\", Default" w234 {
              tunnel: [1.0 ("Value") -1.0 ("Value")] -> w233
              tunnel: [255.0 ("Value") 1.0 ("Value")] -> w232
              tunnel: [128.0 ("Value") 0.0 ("Value")] -> w231
              tunnel: [64.0 ("Value") 0.5 ("Value")] -> w230
              frame "PWM" {
              }
              frame "Motor", Default {
              }
            }
            n129 = property on="Motor" class="Clust (strict)"("Visible"=TRUE) -> ()  [unwired: 2 in, 2 out]
            n130 = property on="Value" class="Slide (strict)"("Value"=w231, "Scale.Minimum"=w233, "Scale.Maximum"=w232, "Scale.Increment"=w230) -> ()  [unwired: 2 in, 2 out]
            n131 = property on="On/Off" class="Bool (strict)"("Visible"=w235) -> ()  [unwired: 2 in, 2 out]
            n132 = property on="Test Slider" class="Slide (strict)"("Visible"=w235) -> ()  [unwired: 2 in, 2 out]
            n133 = property on="Test Ring" class="Ring (strict)"("Visible"=w235) -> ()  [unwired: 2 in, 2 out]
            n134 = property on="Rev/Fwd" class="Clust (strict)"("Visible"=w235) -> ()  [unwired: 2 in, 2 out]
          }
          frame "Servo" {
            w247 = FALSE ("Visible")
            n135 = call <vilib>:"NT Read Number.vi"("Name"=w249) -> ("Numeric"=w248:dbl)  [unwired: 9 in, 1 out]
            n136 = property on="Test Slider" class="Slide (strict)"("Visible"=TRUE, "Scale.Maximum"=170.0 ("Scale.Range:Maximum")) -> ()  [unwired: 2 in, 2 out]
            n137 = local write "Test Slider"(w248) -> ()
            n138 = property on="Motor" class="Clust (strict)"("Visible"=w247) -> ()  [unwired: 2 in, 2 out]
            n139 = property on="Rev/Fwd" class="Clust (strict)"("Visible"=w247) -> ()  [unwired: 2 in, 2 out]
            n140 = property on="On/Off" class="Bool (strict)"("Visible"=w247) -> ()  [unwired: 2 in, 2 out]
            n141 = property on="Test Ring" class="Ring (strict)"("Visible"=w247) -> ()  [unwired: 2 in, 2 out]
          }
          frame "Relay", "Solenoid" {
            w250 = FALSE ("Visible")
            n142 = property on="Motor" class="Clust (strict)"("Visible"=w250) -> ()  [unwired: 2 in, 2 out]
            n143 = property on="Test Slider" class="Slide (strict)"("Visible"=w250) -> ()  [unwired: 2 in, 2 out]
            n144 = Search and Replace String(input string=w251, search string="/Value  **", replace string="/Direction") -> (result string=w257:string)  [unwired: 5 in, 3 out]
            n145 = property on="Test Ring" class="Ring (strict)"("Visible"=w250) -> ()  [unwired: 2 in, 2 out]
            n146 = call <vilib>:"NT Read String.vi"("Name"=w257) -> ("String"=w255:string)  [unwired: 9 in, 1 out]
            n147 = Equal?(x="Both directions", y=w255) -> (x = y?=w253:bool)
            n148 = Not(x=w253) -> (.not. x?=w254:bool)
            n149 = property on="Rev/Fwd" class="Clust (strict)"("Visible"=w253) -> ()  [unwired: 2 in, 2 out]
            n150 = property on="On/Off" class="Bool (strict)"("Visible"=w254, "Caption.Text"=w252) -> ()  [unwired: 2 in, 2 out]
          }
          frame "Compressor", "Digital Out" {
            w260 = FALSE ("Visible")
            # "Get direction and finish"
            n151 = property on="Motor" class="Clust (strict)"("Visible"=w260) -> ()  [unwired: 2 in, 2 out]
            n152 = property on="Test Slider" class="Slide (strict)"("Visible"=w260) -> ()  [unwired: 2 in, 2 out]
            n153 = property on="Test Ring" class="Ring (strict)"("Visible"=w260) -> ()  [unwired: 2 in, 2 out]
            n154 = property on="On/Off" class="Bool (strict)"("Visible"=TRUE, "Caption.Text"=w261) -> ()  [unwired: 2 in, 2 out]
            n155 = property on="Rev/Fwd" class="Clust (strict)"("Visible"=FALSE) -> ()  [unwired: 2 in, 2 out]
          }
          frame "Camera" {
            n156 = call <vilib>:"Get Last Path Segment.vi"("String in"=w268) -> ("String out"=w269:string)  [unwired: 10 in]
            n157 = property on="On/Off" class="Bool (strict)"("Visible"=FALSE) -> ()  [unwired: 2 in, 2 out]
            n158 = property on="Motor" class="Clust (strict)"("Visible"=FALSE) -> ()  [unwired: 2 in, 2 out]
            n159 = property on="Rev/Fwd" class="Clust (strict)"("Visible"=FALSE) -> ()  [unwired: 2 in, 2 out]
            n160 = case shown="\"White Balance  **\"" w269 {
              tunnel: w268 -> [w275 w284 w293 w302 w311 _ w317]
              tunnel: w267 -> [w273 w281 w290 w299 w308 _ _]
              frame "Size  **" {
                n161 = Index Array(array=w273) -> (element=w272:cluster{string[]})  [unwired: 1 in]
                n162 = call <vilib>:"NT Read String.vi"("Name"=w275) -> ("String"=w274:string)  [unwired: 9 in, 1 out]
                n163 = Unbundle(w272) -> (w270:string[])
                n164 = Match First String(2:w270, 3:w274) -> (0:w271:i32)  [unwired: 1 out]
                n165 = property on="Test Ring" class="Ring (strict)"("Value"=w271, "Strings []"=w270) -> ()  [unwired: 2 in, 2 out]
                n166 = property on="Test Ring" class="Ring (strict)"("Visible"=TRUE) -> ()  [unwired: 2 in, 2 out]
                n167 = property on="Test Slider" class="Slide (strict)"("Visible"=FALSE) -> ()  [unwired: 2 in, 2 out]
              }
              frame "White Balance  **" {
                n168 = Index Array(array=w281, index=1) -> (element=w282:cluster{string[]})
                n169 = call <vilib>:"NT Read String.vi"("Name"=w284) -> ("String"=w283:string)  [unwired: 9 in, 1 out]
                n170 = Unbundle(w282) -> (w279:string[])
                n171 = Match First String(2:w279, 3:w283) -> (0:w278:i32)  [unwired: 1 out]
                n172 = property on="Test Ring" class="Ring (strict)"("Value"=w278, "Strings []"=w279) -> ()  [unwired: 2 in, 2 out]
                n173 = property on="Test Ring" class="Ring (strict)"("Visible"=TRUE) -> ()  [unwired: 2 in, 2 out]
                n174 = property on="Test Slider" class="Slide (strict)"("Visible"=FALSE) -> ()  [unwired: 2 in, 2 out]
              }
              frame "Exposure  **" {
                n175 = Index Array(array=w290, index=2) -> (element=w291:cluster{string[]})
                n176 = call <vilib>:"NT Read String.vi"("Name"=w293) -> ("String"=w292:string)  [unwired: 9 in, 1 out]
                n177 = Unbundle(w291) -> (w287:string[])
                n178 = Match First String(2:w287, 3:w292) -> (0:w288:i32)  [unwired: 1 out]
                n179 = property on="Test Ring" class="Ring (strict)"("Value"=w288, "Strings []"=w287) -> ()  [unwired: 2 in, 2 out]
                n180 = property on="Test Ring" class="Ring (strict)"("Visible"=TRUE) -> ()  [unwired: 2 in, 2 out]
                n181 = property on="Test Slider" class="Slide (strict)"("Visible"=FALSE) -> ()  [unwired: 2 in, 2 out]
              }
              frame "Exposure Priority  **" {
                n182 = Index Array(array=w299, index=3) -> (element=w300:cluster{string[]})
                n183 = call <vilib>:"NT Read String.vi"("Name"=w302) -> ("String"=w301:string)  [unwired: 9 in, 1 out]
                n184 = Unbundle(w300) -> (w296:string[])
                n185 = Match First String(2:w296, 3:w301) -> (0:w297:i32)  [unwired: 1 out]
                n186 = property on="Test Ring" class="Ring (strict)"("Value"=w297, "Strings []"=w296) -> ()  [unwired: 2 in, 2 out]
                n187 = property on="Test Ring" class="Ring (strict)"("Visible"=TRUE) -> ()  [unwired: 2 in, 2 out]
                n188 = property on="Test Slider" class="Slide (strict)"("Visible"=FALSE) -> ()  [unwired: 2 in, 2 out]
              }
              frame "Color Enable  **" {
                n189 = Index Array(array=w308, index=4) -> (element=w309:cluster{string[]})
                n190 = call <vilib>:"NT Read String.vi"("Name"=w311) -> ("String"=w310:string)  [unwired: 9 in, 1 out]
                n191 = Unbundle(w309) -> (w305:string[])
                n192 = Match First String(2:w305, 3:w310) -> (0:w306:i32)  [unwired: 1 out]
                n193 = property on="Test Ring" class="Ring (strict)"("Value"=w306, "Strings []"=w305) -> ()  [unwired: 2 in, 2 out]
                n194 = property on="Test Ring" class="Ring (strict)"("Visible"=TRUE) -> ()  [unwired: 2 in, 2 out]
                n195 = property on="Test Slider" class="Slide (strict)"("Visible"=FALSE) -> ()  [unwired: 2 in, 2 out]
              }
              frame Default {
                n196 = property on="Test Ring" class="Ring (strict)"("Visible"=FALSE) -> ()  [unwired: 2 in, 2 out]
                n197 = property on="Test Slider" class="Slide (strict)"("Visible"=FALSE) -> ()  [unwired: 2 in, 2 out]
              }
              frame "Brightness  **", "Color Level  **", "Compression  **", "FPS  **", "Sharpness  **" {
                n198 = call <vilib>:"NT Read Number.vi"("Name"=w317) -> ("Numeric"=w316:dbl)  [unwired: 9 in, 1 out]
                n199 = local write "Test Slider"(w316) -> ()
                n200 = property on="Test Slider" class="Slide (strict)"("Visible"=TRUE, "Scale.Maximum"=100.0 ("Scale.Range:Maximum")) -> ()  [unwired: 2 in, 2 out]
                n201 = property on="Test Ring" class="Ring (strict)"("Visible"=FALSE) -> ()  [unwired: 2 in, 2 out]
              }
            }
          }
        }
        n202 = property on="Progress" class="Clust (strict)"("Visible"=FALSE) -> ()  [unwired: 2 in, 2 out]
      }
      event "Test Name": Mouse Enter {
        # "Populate the ring with the list of tests"
        n203 = event-data() -> ()  [unwired: 1 in, 1 out]
        n204 = call <vilib>:"NT Read String Array.vi"("Name"="TestMode/TestList") -> ("String Array"=w325:string[])  [unwired: 9 in, 1 out]
        n205 = Build Array (concatenate)("Select the test to run...", w325) -> (w324:string[])
        n206 = property on="Test Name" class="Ring (strict)"("Strings []"=w324) -> ()  [unwired: 2 in, 2 out]
      }
      event "Test Name": Value Change {
        w327 = FALSE ("Visible")
        # "Tell the robot the test name to run"
        n207 = event-data() -> ("NewVal"=w331:u16)  [unwired: 1 in]
        n208 = property on="Test Name" class="Ring (strict)"() -> ("Strings []"=w332:string[])  [unwired: 2 in, 2 out]
        n209 = local write "Progress"(T9 {"Test Progress"=0, "Test Progress Text"=""} ("Progress")) -> ()
        n210 = Index Array(array=w332, index=w331) -> (element=w330:string)
        n211 = call <vilib>:"NT Write String.vi"("String"=w330, "Name"="TestMode/TestName") -> ()  [unwired: 9 in, 1 out]
        n212 = property on="Progress" class="Clust (strict)"("Visible"=TRUE) -> ()  [unwired: 2 in, 2 out]
        n213 = property on="Motor" class="Clust (strict)"("Visible"=w327) -> ()  [unwired: 2 in, 2 out]
        n214 = property on="Test Slider" class="Slide (strict)"("Visible"=w327) -> ()  [unwired: 2 in, 2 out]
        n215 = property on="On/Off" class="Bool (strict)"("Visible"=w327) -> ()  [unwired: 2 in, 2 out]
        n216 = property on="Rev/Fwd" class="Clust (strict)"("Visible"=w327) -> ()  [unwired: 2 in, 2 out]
        n217 = property on="Test Ring" class="Ring (strict)"("Visible"=w327) -> ()  [unwired: 2 in, 2 out]
      }
      event "Listbox": Double Click {
        # "Shift clears all"
        # "Update symbols on the listbox"
        n218 = event-data() -> ("PlatMods.Shift"=w335:bool, "Row"=w337:i32)  [unwired: 1 in]
        n219 = case shown="True" w335 {
          tunnel: w337 -> [w341 _]
          tunnel: 1 -> [w340 _]
          frame False {
            n220 = property on="Listbox" class="LstBox (strict)"() -> ("Item Symbols"=w339:i32[])  [unwired: 2 in, 2 out]
            n221 = Replace Array Subset(array=w339, new element=w340, index=w341) -> (w338:i32[])
            n222 = property on="Listbox" class="LstBox (strict)"("Item Symbols"=w338) -> ()  [unwired: 2 in, 2 out]
          }
          frame True {
            w342 = 0 ("Top Row")
            n223 = property on="Listbox" class="LstBox (strict)"() -> ("Number of Rows"=w344:u32)  [unwired: 2 in, 2 out]
            n224 = Initialize Array(0, w344) -> (w343:i32[])
            n225 = property on="Listbox" class="LstBox (strict)"("Top Row"=w342, "Value"=w342, "Item Symbols"=w343) -> ()  [unwired: 2 in, 2 out]
          }
        }
      }
      event "Listbox": Key Down {
        # "Update symbols on the listbox\nLeft and right keys check and uncheck"
        n226 = event-data() -> ("VKey"=w348:T24)  [unwired: 1 in]
        n227 = case shown="\"Left\", \"Right\"" w348 {
          selector: w348 -> [w353 _]
          tunnel: eventvkey."Left" ("VKey") -> [w351 _]
          frame "Left", "Right" {
            n228 = Equal?(x=w351, y=w353) -> (x = y?=w352:bool)
            n229 = Select(t=0, s=w352, f=1) -> (s? t:f=w354:i32)
            n230 = property on="Listbox" class="LstBox (strict)"() -> ("Item Symbols"=w357:i32[])  [unwired: 2 in, 2 out]
            n231 = Replace Array Subset(array=w357, new element=w354, index="Listbox") -> (w356:i32[])
            n232 = property on="Listbox" class="LstBox (strict)"("Item Symbols"=w356) -> ()  [unwired: 2 in, 2 out]
          }
          frame Default {
          }
        }
      }
      event "DB Camera Config": Value Change {
        # "Show or hide the cluster of controls, store in ini file"
        n233 = event-data() -> ("NewVal"=w361:bool)  [unwired: 1 in]
        n234 = case shown="False" w361 {
          tunnel: w360 -> [w370 _]
          tunnel: [w363 w381] -> w359
          tunnel: w358 -> [w362 w381]
          frame False {
            w377 = "Camera"
            w380 = FALSE ("Visible")
            n235 = local read "Camera Settings"() -> (w369:T2)
            n236 = Index Array(array=w370) -> (element=w373:cluster{string[]})  [unwired: 1 in]
            n237 = Unbundle(w369) -> ("Frame Rate"=w368:i32, "Compression"=w367:i32, "Size"=w371:u16)
            n238 = Unbundle(w373) -> (w372:string[])
            n239 = Index Array(array=w372, index=w371) -> (element=w366:string)
            n240 = call-poly <vilib>:"Write Key.vi"("section"=w377, "value"=w366, "key"="Size", "refnum"=w362) -> ("refnum out"=w379:T22)  [unwired: 2 in, 5 out]
            n241 = call-poly <vilib>:"Write Key.vi"("section"=w377, "value"=w368, "key"="FrameRate", "refnum"=w379) -> ("refnum out"=w378:T22)  [unwired: 1 in, 6 out]
            n242 = property on="Camera Settings" class="Clust (strict)"("Visible"=w380) -> ()  [unwired: 2 in, 2 out]
            n243 = local write "DB Camera Config"(w380) -> ()
            n244 = call-poly <vilib>:"Write Key.vi"("section"=w377, "value"=w367, "key"="Compression", "refnum"=w378) -> ("refnum out"=w364:T22)  [unwired: 1 in, 6 out]
            n245 = call <vilib>:"Close Config Data.vi"("refnum"=w364) -> ("file path"=w365:path)  [unwired: 2 in, 8 out]
            n246 = call <vilib>:"Open Config Data.vi"("configuration file path"=w365) -> ("refnum"=w363:T22)  [unwired: 8 in, 2 out]
          }
          frame True {
            n247 = property on="Camera Settings" class="Clust (strict)"("Visible"=TRUE) -> ()  [unwired: 2 in, 2 out]
          }
        }
      }
      event "Camera Settings": Value Change {
        # "Update summary string when any elements of DB camera change"
        n248 = event-data() -> ("NewVal"=w394:T2)  [unwired: 1 in]
        n249 = Index Array(array=w390) -> (element=w389:cluster{string[]})  [unwired: 1 in]
        n250 = Unbundle(w394) -> ("Frame Rate"=w385:i32, "Compression"=w384:i32, "Size"=w387:u16)
        n251 = Unbundle(w389) -> (w388:string[])
        n252 = Index Array(array=w388, index=w387) -> (element=w386:string)
        n253 = Format Into String(format string="%s   %dfps   %d%%", w386, w385, w384) -> (resulting string=w391:string)  [unwired: 2 in, 1 out]
        n254 = Build Array(w391) -> (w392:string[])
        n255 = property on="DB Camera Config" class="Bool (strict)"("Strings [4]"=w392) -> ()  [unwired: 2 in, 2 out]
      }
      event "Motor.Enable": Value Change {
        # "When the test mode otor enable helper is set, update that\ntree row item's value"
        n256 = event-data() -> ("NewVal"=w400:bool)  [unwired: 1 in]
        n257 = Unbundle("Motor") -> ("Value"=w399:dbl)  [unwired: 1 out]
        n258 = Select(t=w399, s=w400, f=0.0) -> (s? t:f=w397:dbl)
        n259 = call <vilib>:"NT Write Number.vi"("Numeric"=w397, "Name"=w396) -> ()  [unwired: 9 in, 1 out]
      }
      event "Test Slider": Value Change {
        # "When the test mode slider helper is set, update that\ntree row item's value"
        n260 = event-data() -> ("NewVal"=w403:dbl)  [unwired: 1 in]
        n261 = call <vilib>:"NT Write Number.vi"("Numeric"=w403, "Name"=w404) -> ()  [unwired: 9 in, 1 out]
      }
      event "On/Off": Value Change {
        # "When the test mode on/off helper value is set, update that\ntree row item's value"
        n262 = event-data() -> ("NewVal"=w408:bool)  [unwired: 1 in]
        n263 = Boolean To (0,1)(Boolean=w408) -> (0, 1=w407:i16)
        n264 = call <vilib>:"NT Write Number.vi"("Numeric"=w407, "Name"=w406) -> ()  [unwired: 9 in, 1 out]
      }
      event "Rev/Fwd": Value Change {
        # "When the test mode helper value for relays is set, update that\ntree row item's value"
        n265 = event-data() -> ("NewVal.Forward"=w416:bool, "NewVal.Reverse"=w415:bool)  [unwired: 1 in]
        n266 = Boolean To (0,1)(Boolean=w416) -> (0, 1=w412:i16)
        n267 = Boolean To (0,1)(Boolean=w415) -> (0, 1=w414:i16)
        n268 = Negate(x=w414) -> (-x=w413:i16)
        n269 = Add(x=w412, y=w413) -> (x+y=w411:i16)
        n270 = call <vilib>:"NT Write Number.vi"("Numeric"=w411, "Name"=w410) -> ()  [unwired: 9 in, 1 out]
      }
      event "Test Ring": Value Change {
        # "When a test mode helper value is selected from the ring,\nset the tree item's variable to the string value"
        n271 = event-data() -> ("NewVal"=w420:u16)  [unwired: 1 in]
        n272 = property on="Test Ring" class="Ring (strict)"() -> ("Strings []"=w421:string[])  [unwired: 2 in, 2 out]
        n273 = Index Array(array=w421, index=w420) -> (element=w419:string)
        n274 = call <vilib>:"NT Write String.vi"("String"=w419, "Name"=w418) -> ()  [unwired: 9 in, 1 out]
      }
      event "Rec Mode": Value Change {
        # "Update globals for recording mode and path to read log from.\nClear when logging and let NetworkTables set path for vision to\nuse."
        n275 = event-data() -> ("NewVal"=w431:enum32{"Stop", "Record", "Playback"})  [unwired: 1 in]
        n276 = global write "WPI_DashboardLogging Global.vi" "Logging Filename"(path "") -> ()
        n277 = case shown="\"Playback\"" w431 {
          tunnel: w430 -> [_ w433 w441]
          tunnel: [_ _ w440] -> w427
          tunnel: [_ _ w439] -> _
          tunnel: w425 -> [_ _ w437]
          tunnel: cluster{i32, i32} {-250, 170} -> [_ _ w436]
          tunnel: [_ _ T25 {"Image Size"=TRUE, "Image Type"=TRUE, "Pixel Value"=TRUE, "ROI Information"=TRUE, "Zoom Factor"=FALSE} ("Image Information Shown:All Elements")] -> w423
          tunnel: [_ _ TRUE ("Zoom Factor")] -> w422
          frame Default {
          }
          frame "Stop", "Record" {
            # "Place Window too"
            n278 = invoke class="VI" method="FP.Close"(reference=w433) -> (reference out=w432:refnum<vi>)  [unwired: 2 in, 2 out]
            n279 = invoke class="VI" method="Abort VI"(reference=w432) -> ()  [unwired: 2 in, 3 out]
          }
          frame "Playback" {
            n280 = call "Open Playback Panel.vi"("Offset"=w436, "DB VI Ref"=w437, "Playback in"=w441) -> ("Playback out"=w438:refnum<vi>)  [unwired: 8 in]
            n281 = register-events(w438) -> (reference out=w440:refnum<event-registration>, error out=w439:errorcluster)  [unwired: 2 in]
          }
        }
        n282 = global write "WPI_DashboardLogging Global.vi" "Recording"(w431) -> ()
        n283 = property on="Camera Image" class="ImageControl"("Image Information Shown"=w423, "Image Information Visible"=w422) -> ()  [unwired: 2 in, 2 out]
        n284 = call <vilib>:"WPI_DashboardNT Log FieldName Cache.vi"("Operation"=enum16{"Lookup/Add", "Index", "Clear"}."Clear") -> ()  [unwired: 8 in, 3 out]
      }
      event Panel Close {
        w442 = enum32{"Stop", "Record", "Playback"}."Stop" ("Rec Mode")
        # "Playback window has been closed, abort"
        n285 = event-data() -> ()  [unwired: 1 in, 4 out]
        n286 = local write "Rec Mode"(w442) -> ()
        n287 = global write "WPI_DashboardLogging Global.vi" "Recording"(w442) -> ()
      }
      event Panel Close {
        # "Abort playback window and ourself"
        n288 = event-data() -> ()  [unwired: 1 in, 4 out]
        n289 = invoke class="VI" method="FP.Close"(reference=w447) -> (reference out=w446:refnum<vi>)  [unwired: 2 in, 2 out]
        n290 = invoke class="VI" method="Abort VI"(reference=w446) -> (error out=w445:errorcluster)  [unwired: 2 in, 2 out]
        n291 = invoke class="VI" method="Abort VI"(error in=w445) -> ()  [unwired: 2 in, 3 out]
      }
      event "Vision": Value Change {
        # "Enable/Disable Compression slider.\nHW USB is hard-coded into the camera"
        n292 = event-data() -> ("NewVal"=w453:u16)  [unwired: 1 in]
        n293 = Equal?(x=w453, y=u32 2 ("milliseconds to wait")) -> (x = y?=w451:bool)
        n294 = Select(t=T26."Disabled and Grayed Out" ("Disabled"), s=w451, f=T26."Enabled" ("Disabled")) -> (s? t:f=w448:T26)
        n295 = property on="Compression" class="Slide (strict)"("DisabledEnum"=w448) -> ()  [unwired: 2 in, 2 out]
      }
    }
  }
  n296 = while {
    tunnel: w37 -> [w456]
    i -> [w459]
    stop <- FALSE stop-if-true
    n297 = Wait (ms)(milliseconds to wait=u32 100) -> ()  [unwired: 1 out]
    n298 = case shown="\"Playback\"" "Rec Mode" {
      tunnel: w459 -> [_ _ w474]
      tunnel: [u32 2829099 ("Base Color") u32 11141120 ("Target Color") w463] -> w455
      frame "Stop", Default {
        # "Reset the color, extra updates don't cost much"
      }
      frame "Record" {
      }
      frame "Playback" {
        # "Playback"
        n299 = Quotient & Remainder(x=w474, y=u32 50 ("milliseconds to wait")) -> (x-y*floor(x/y)=w470:u32)  [unwired: 1 out]
        n300 = Divide(x=w470, y=u32 50 ("milliseconds to wait")) -> (x/y=w467:dbl)
        n301 = Multiply(x=6.283185307179586, y=w467) -> (x*y=w472:dbl)
        n302 = Sine(x=w472) -> (sin(x)=w471:dbl)
        n303 = Absolute Value(x=w471) -> (abs(x)=w464:dbl)
        n304 = call "Interpolate RGB Color.vi"("Proportion"=w464, "Target Color"=u32 30976, "Base Color"=u32 2829099) -> ("Result Color"=w463:u32)  [unwired: 8 in]
      }
    }
    n305 = property class="Pane"(reference=w456, "PaneColor"=w455) -> ()  [unwired: 1 in, 2 out]
  }
  n306 = disable-structure shown="Disabled" {
    frame Disabled {
      # "Loop 7. Wait for DS connections"
      n307 = TCP Create Listener(10:u16 1741 ("timeout ms (25000)")) -> (3:w475:refnum<k5>)  [unwired: 4 in, 2 out]
      n308 = while {
        tunnel: w475 -> [w478]
        stop <- FALSE stop-if-true
        n309 = TCP Wait On Listener(11:w478) -> (4:w477:refnum<k5>)  [unwired: 3 in, 4 out]
        n310 = local write "TCP"(w477) -> ()
      }
    }
    frame Enabled {
    }
  }
  n311 = while {
    tunnel: u16 1741 ("timeout ms (25000)") -> [w483]
    stop <- FALSE stop-if-true
    n312 = TCP Create Listener(10:w483) -> (0:w482:errorcluster, 3:w481:refnum<k5>)  [unwired: 4 in, 1 out]
    n313 = case shown="No Error" w482 {
      selector: w482 -> [w484 _]
      tunnel: w481 -> [w485 _]
      frame No Error {
        n314 = while {
          tunnel: w485 -> [w490]
          tunnel: w484 -> [w486]
          stop <- FALSE stop-if-true
          n315 = TCP Wait On Listener(8:w486, 11:w490) -> (0:w488:errorcluster, 4:w489:refnum<k5>)  [unwired: 2 in, 3 out]
          n316 = case shown="Error" w488 {
            frame No Error {
            }
            frame Error {
              n317 = Wait (ms)(milliseconds to wait=u32 100) -> ()  [unwired: 1 out]
            }
          }
          n318 = local write "TCP"(w489) -> ()
        }
      }
      frame Error {
      }
    }
  }
  n319 = property on="On/Off" class="Bool (strict)"("Visible"=w5) -> ()  [unwired: 2 in, 2 out]
  n320 = property on="Motor" class="Clust (strict)"("Visible"=w5) -> ()  [unwired: 2 in, 2 out]
  n321 = property on="Progress" class="Clust (strict)"("Visible"=w5) -> ()  [unwired: 2 in, 2 out]
  n322 = property on="Test Ring" class="Ring (strict)"("Visible"=w5) -> ()  [unwired: 2 in, 2 out]
  n323 = property on="Rev/Fwd" class="Clust (strict)"("Visible"=w5) -> ()  [unwired: 2 in, 2 out]
  n324 = property on="Camera Settings" class="Clust (strict)"("Visible"=w5) -> ()  [unwired: 2 in, 2 out]
  n325 = local write "DB Camera Config"(w5) -> ()
  n326 = global write "WPI_DashboardLogging Global.vi" "Recording"(w31) -> ()
  n327 = local write "Rec Mode"(w31) -> ()
